vi "Read Target Address.vi"(8 "error in (no error)":errorcluster, 11 "Address in":refnum<class "Address.lvclass">) -> (0 "error out":errorcluster, 2 "Target Address":i16 format="%.0x", 3 "Address out":refnum<class "Address.lvclass">)   [LabVIEW 2020, in "Address.lvclass"]
uses:
  Address.lvclass
  Address.lvclass/Address.ctl
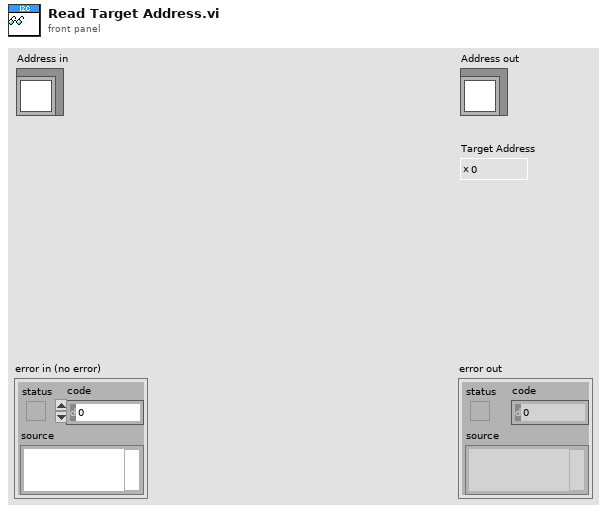
[diagram p1: front panel]
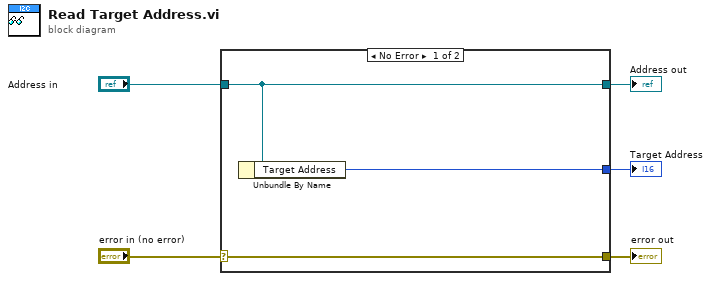
[diagram p0: block diagram]
diagram:
  n1 = case shown="No Error" "error in (no error)" {
    selector: "error in (no error)" -> [w8 w9]
    tunnel: [w8 w9] -> w4
    tunnel: [w7 w10] -> w2
    tunnel: "Address in" -> [w7 w10]
    tunnel: [w6 _] -> w1
    frame No Error {
      n2 = Unbundle By Name(w7) -> ("Target Address"=w6:i16)
    }
    frame Error {
    }
  }
  "error out" <- w4
  "Address out" <- w2
  "Target Address" <- w1
